vi "set_parameter.vi"(8 "error in (no error)":errorcluster, 10 "parameter":string, 11 "result in":refnum<class "result.lvclass">) -> (0 "error out":errorcluster, 3 "result out":refnum<class "result.lvclass">)   [LabVIEW 2015, in "result.lvclass"]
uses:
  result.lvclass
  result.lvclass/result.ctl
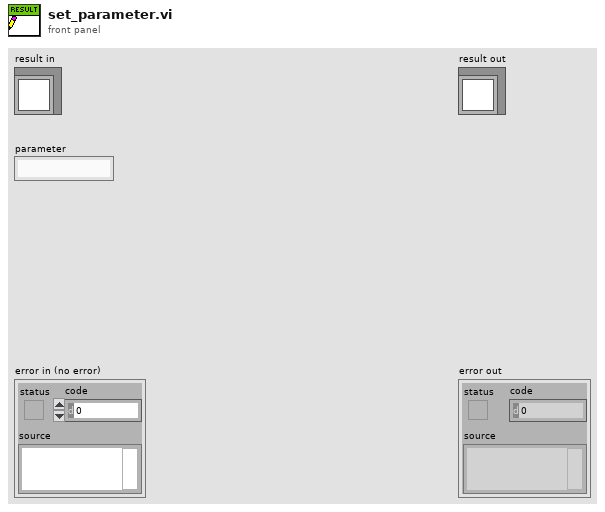
[diagram p1: front panel]
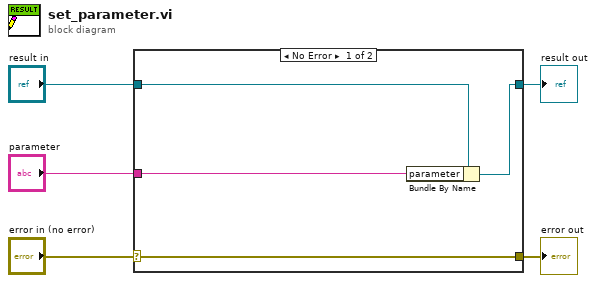
[diagram p0: block diagram]
diagram:
  n1 = case shown="No Error" "error in (no error)" {
    selector: "error in (no error)" -> [w9 w10]
    tunnel: [w9 w10] -> w4
    tunnel: [w7 w11] -> w2
    tunnel: "result in" -> [w8 w11]
    tunnel: "parameter" -> [w6 _]
    frame No Error {
      n2 = Bundle By Name(cluster=w8, "parameter"=w6) -> (w7:refnum<class "result.lvclass">)
    }
    frame Error {
    }
  }
  "error out" <- w4
  "result out" <- w2
